vi "PROVA-HV-ILEAK.vi"() -> ()   [LabVIEW 2015]
uses:
  dr_Keithley 24XX/Keithley 24XX.lvlib
  VIPM2.lvlib
panel:
  out "Timestamp":sgl[](array[numeric])
  out "barra":u8(slide) scale=0.0..5.0
  in  "Abort":bool
  in  "VISA resource name":refnum<visa-resource-name>="GPIB1::25::INSTR"
  out "Current":sgl format="%#_6p"
  out "Voltage":sgl
  out "Chart":cluster{sgl, sgl}[](graph)
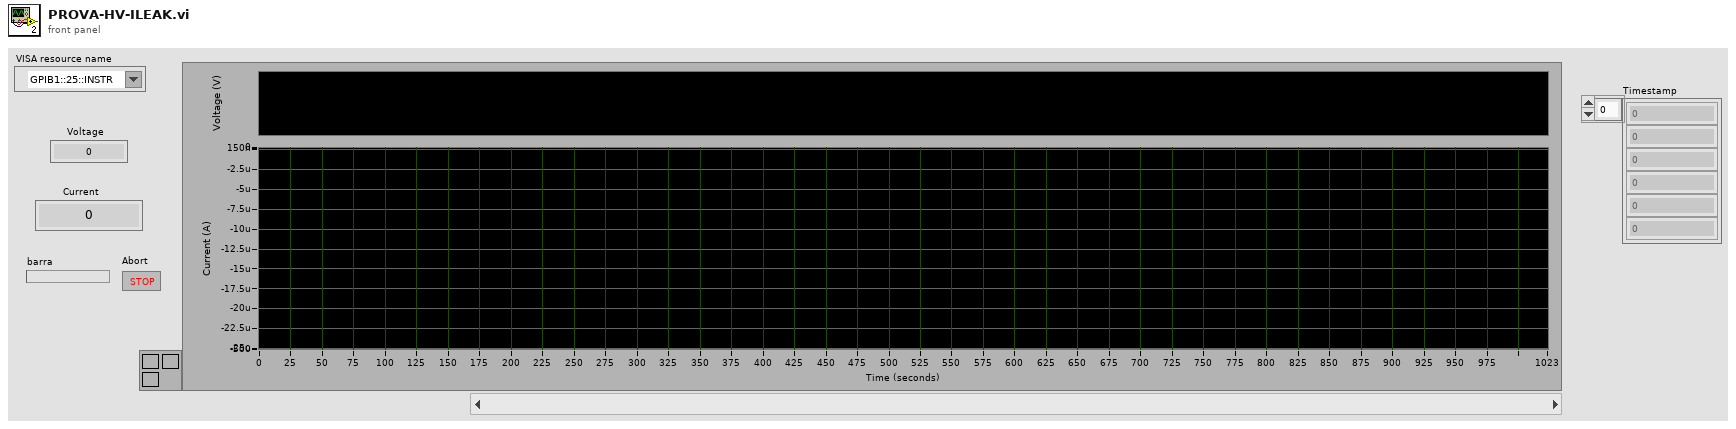
[diagram p1: front panel]
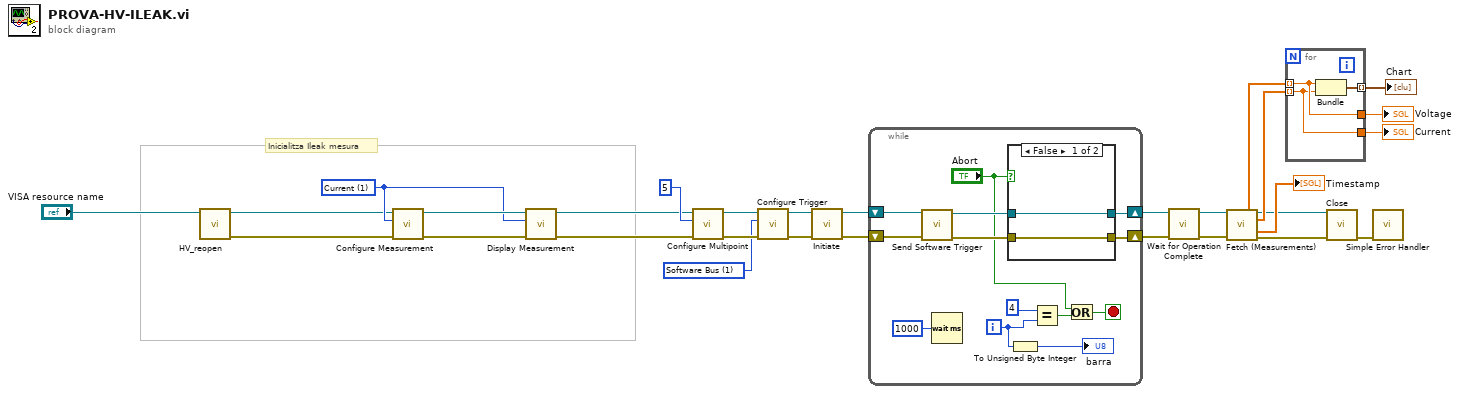
[diagram p0: block diagram]
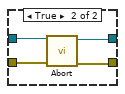
[diagram p2: hidden frame]
diagram:
  w11 = u16 1 items=["Volts", "Current", "Resistance"] ("Function (0: Volts)")
  w26 = u16 1 items=["Immediate", "Software Bus", "Timer", "Manual", "Trigger Link", "Rising SOT Pulse", "Falling SOT Pulse", "Rising or Falling SOT Pulse"] ("Arming Source  (0: Immediate)")
  # "Inicialitza Ileak mesura"
  n1 = call "HV_reopen.vi"("VISA resource name"="VISA resource name") -> ("error out"=w5:errorcluster, "VISA resource name out"=w4:refnum<visa-resource-name>)  [unwired: 9 in]
  n2 = call "Configure Measurement.vi"("error in (no error)"=w5, "Function (0: Volts)"=w11, "VISA resource name"=w4) -> ("error out"=w12:errorcluster, "VISA resource name out"=w13:refnum<visa-resource-name>)  [unwired: 7 in]
  n3 = call "Display Measurement.vi"("error in (no error)"=w12, "Displayed Measurement (0: Voltage)"=w11, "VISA resource name"=w13) -> ("error out"=w10:errorcluster, "VISA resource name out"=w9:refnum<visa-resource-name>)  [unwired: 7 in]
  n4 = call "Configure Multipoint.vi"("error in (no error)"=w10, "Number of Times to Arm (1)"=5 ("Trigger Count (1)"), "VISA resource name"=w9) -> ("error out"=w27:errorcluster, "VISA resource name out"=w28:refnum<visa-resource-name>)  [unwired: 7 in]
  n5 = call "Configure Trigger.vi"("error in (no error)"=w27, "Arming Source  (0: Immediate)"=w26, "VISA resource name"=w28) -> ("error out"=w24:errorcluster, "VISA resource name out"=w25:refnum<visa-resource-name>)  [unwired: 7 in]
  n6 = call "Initiate.vi"("error in (no error)"=w24, "VISA resource name"=w25) -> ("error out"=w22:errorcluster, "VISA resource name out"=w23:refnum<visa-resource-name>)  [unwired: 8 in]
  n7 = while {
    shift-right: [w35] -> w21
    shift-left: w23 -> [w41]
    shift-right: [w34] -> w20
    shift-left: w22 -> [w40]
    i -> [w31]
    stop <- w38 stop-if-true
    n8 = call "Send Software Trigger.vi"("error in (no error)"=w40, "VISA resource name"=w41) -> ("error out"=w36:errorcluster, "VISA resource name out"=w37:refnum<visa-resource-name>)  [unwired: 8 in]
    n9 = Wait (ms)(milliseconds to wait=u32 1000 ("millisecond multiple")) -> ()  [unwired: 1 out]
    n10 = case shown="False" "Abort" {
      tunnel: w37 -> [w44 w48]
      tunnel: w36 -> [w43 w46]
      tunnel: [w44 w47] -> w35
      tunnel: [w43 w45] -> w34
      frame False {
      }
      frame True {
        n11 = call "Abort.vi"("error in (no error)"=w46, "VISA resource name"=w48) -> ("error out"=w45:errorcluster, "VISA resource name out"=w47:refnum<visa-resource-name>)  [unwired: 8 in]
      }
    }
    n12 = To Unsigned Byte Integer(number=w31) -> (unsigned 8bit integer=→"barra":u8)
    n13 = Equal?(x=4 ("y"), y=w31) -> (x = y?=w39:bool)
    n14 = Or(x="Abort", y=w39) -> (x .or. y?=w38:bool)
  }
  n15 = call "Wait for Operation Complete.vi"("error in (no error)"=w20, "VISA resource name"=w21) -> ("error out"=w18:errorcluster, "VISA resource name out"=w19:refnum<visa-resource-name>)  [unwired: 8 in]
  n16 = call "Fetch (Measurements).vi"("VISA resource name"=w19, "error in (no error)"=w18) -> ("Voltage"=w16:sgl[], "VISA resource name out"=w2:refnum<visa-resource-name>, "Current"=w15:sgl[], "Timestamp"=→"Timestamp":sgl[], "error out"=w1:errorcluster)  [unwired: 7 in, 2 out]
  n17 = for {
    tunnel: w16 -> [w50] mode=indexing
    tunnel: w15 -> [w49] mode=indexing
    tunnel: [w51] -> w14 mode=indexing
    tunnel: [w50] -> w8
    tunnel: [w49] -> w7
    n18 = Bundle(w50, w49) -> (w51:cluster{sgl, sgl})  [unwired: 1 in]
  }
  "Chart" <- w14
  "Voltage" <- w8
  "Current" <- w7
  n19 = call "Close.vi"("error in (no error)"=w1, "VISA resource name"=w2) -> ("error out"=w29:errorcluster)  [unwired: 9 in]
  n20 = call <vilib>:"Simple Error Handler.vi"("error in (no error)"=w29) -> ()  [unwired: 4 in, 5 out]
